vi "F Dwf Digital Out Status.vi"(8 "error in (no error)":errorcluster, 11 "hdwf":i32) -> (0 "error out":errorcluster, 1 "psts":u8, 3 "function return":i32)   [LabVIEW 2021, in "Olasdwf.lvlib"]
doc: "DWFAPI int FDwfDigitalOutStatus(HDWF hdwf, DwfState *psts);"
uses:
  Olasdwf.lvlib
  Windows/System32/dwf.dll
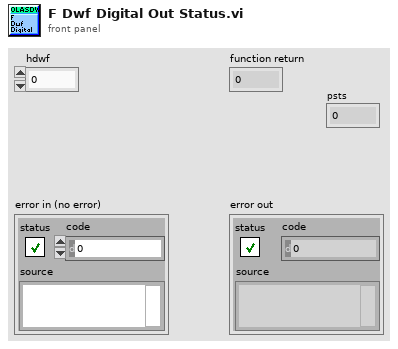
[diagram p1: front panel]
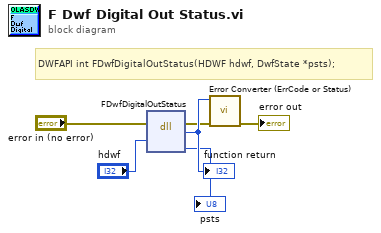
[diagram p0: block diagram]
diagram:
  # "DWFAPI int FDwfDigitalOutStatus(HDWF hdwf, DwfState *psts);"
  n1 = dll-call lib="/Windows/System32/dwf.*" fn="FDwfDigitalOutStatus"(error in="error in (no error)", "hdwf"="hdwf") -> (error out=w3:errorcluster, "return type"=w6:i32, "psts"=→"psts":u8)  [unwired: 4 in, 1 out]
  "function return" <- w6
  n2 = call "Error Converter (ErrCode or Status).vi"("error in (no error)"=w3, "error code"=w6) -> ("error out"=→"error out":errorcluster)  [unwired: 9 in]
